vi "ExperimentLoop.vi"(8 "Error In":errorcluster, 9 "ABLE Configuration":T1, 10 "ABLE Data Structures":T7, 11 "Action Queues":T8) -> (0 "Error Out":errorcluster)   [LabVIEW 2012]
uses:
  ActionQueues.ctl
  UIActionQueueElement.ctl
  UIAction.ctl
  HardwareActionQueueElement.ctl
  HardwareAction.ctl
  ExperimentActionQueueElement.ctl
  ExperimentAction.ctl
  AlarmQueueElement.ctl
  AlarmAction.ctl
  ABLEDataStructures.ctl
  HardwareDisplayData.ctl
  BPM.ctl
  ExperimentHardwareData.ctl
  ExperimentData.ctl
  AlarmData.ctl
  AlarmDatum.ctl
  ABLEConfiguration.ctl
  DisplayConfiguration.ctl
  FolderConfiguration.ctl
  AlarmsConfiguration.ctl
  Keithley6485Configuration.ctl
  Keithley6482Configuration.ctl
  Experiment.ctl
  Sample.ctl
  BeamLine.ctl
  BeamLineType.ctl
  BeamLineIon.ctl
  ExperimentRun.ctl
  ExperimentRunTiming.ctl
  ExperimentRunDose.ctl
  ExperimentRunFluence.ctl
  ExperimentRunTotalCharge.ctl
  ExperimentLogActionQueueElement.ctl
  ExperimentLogAction.ctl
  ExperimentLogData.ctl
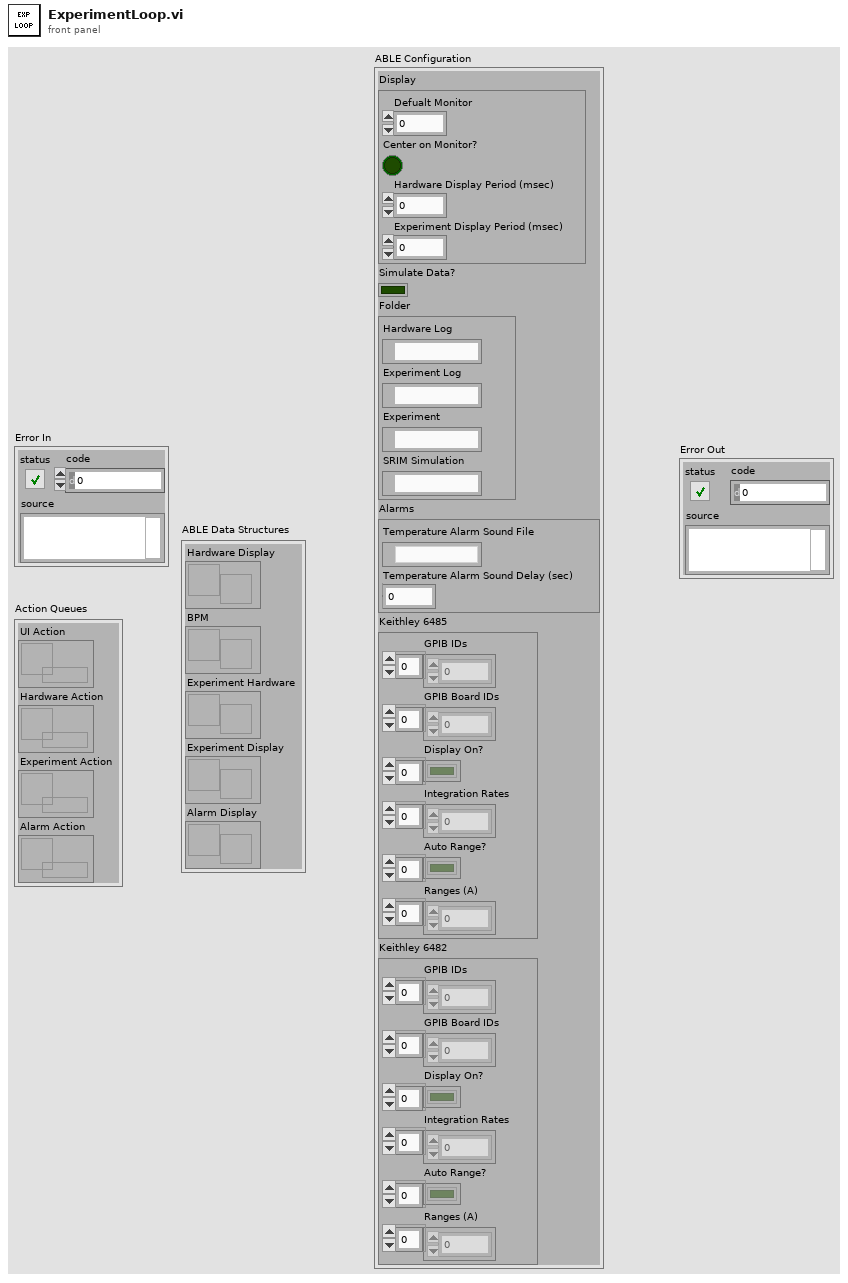
[diagram p1: front panel]
types:
  T1 = typedef "ABLEConfiguration.ctl" = cluster{"Display":T2, "Simulate Data?":bool, "Folder":T3, "Alarms":T4, "Keithley 6485":T5, "Keithley 6482":T6}
  T2 = typedef "DisplayConfiguration.ctl" = cluster{"Defualt Monitor":u16, "Center on Monitor?":bool, "Hardware Display Period (msec)":u32, "Experiment Display Period (msec)":u32}
  T3 = typedef "FolderConfiguration.ctl" = cluster{"Hardware Log":path, "Experiment Log":path, "Experiment":path, "SRIM Simulation":path}
  T4 = typedef "AlarmsConfiguration.ctl" = cluster{"Temperature Alarm Sound File":path, "Temperature Alarm Sound Delay (sec)":dbl}
  T5 = typedef "Keithley6485Configuration.ctl" = cluster{"GPIB IDs":u8[], "GPIB Board IDs":u8[], "Display On?":bool[], "Integration Rates":dbl[], "Auto Range?":bool[], "Ranges (A)":dbl[]}
  T6 = typedef "Keithley6482Configuration.ctl" = cluster{"GPIB IDs":u8[], "GPIB Board IDs":u8[], "Display On?":bool[], "Integration Rates":dbl[], "Auto Range?":bool[], "Ranges (A)":dbl[]}
  T7 = typedef "ABLEDataStructures.ctl" = cluster{"Hardware Display":refnum<notifier>, "BPM":refnum<notifier>, "Experiment Hardware":refnum<notifier>, "Experiment Display":refnum<notifier>, "Alarm Display":refnum<notifier>}
  T8 = typedef "ActionQueues.ctl" = cluster{"UI Action":refnum<queue>, "Hardware Action":refnum<queue>, "Experiment Action":refnum<queue>, "Alarm Action":refnum<queue>}
  T9 = typedef "Experiment.ctl" = cluster{"File Path":path, "Operator":string, "Project":string, "Target Dose (dpa)":dbl, "Sample":T10, "Beam Line":T11, "Runs":T14[]}
  T10 = typedef "Sample.ctl" = cluster{"Name":string, "Description":string, "Molar Mass (g/mol)":dbl, "Density (g/cm^3)":dbl, "Irradiation Area (cm^2)":dbl, "SRIM Damage Peak (disp * ions/cm)":dbl}
  T11 = typedef "BeamLine.ctl" = cluster{"Type":T12, "Ion":T13, "Charge State":u8, "Total Source Ion Energy (kV)":dbl}
  T12 = typedef "BeamLineType.ctl" = enum16{"Ion Beam Analysis", "Auxiliary", "Radiation Damage"}
  T13 = typedef "BeamLineIon.ctl" = enum16{"H", "He", "C", "Fe", "Ni", "Pt", "Si", "Ag", "Au"}
  T14 = typedef "ExperimentRun.ctl" = cluster{"Timing":T15, "Dose (dpa)":T16, "Fluence (ions/cm^2)":T17, "Total Charge (C)":T18}
  T15 = typedef "ExperimentRunTiming.ctl" = cluster{"Start":timestamp, "Stop":timestamp}
  T16 = typedef "ExperimentRunDose.ctl" = cluster{"Start":dbl, "Stop":dbl}
  T17 = typedef "ExperimentRunFluence.ctl" = cluster{"Start":dbl, "Stop":dbl}
  T18 = typedef "ExperimentRunTotalCharge.ctl" = cluster{"Start":dbl, "Stop":dbl}
  T19 = typedef "ExperimentLogData.ctl" = cluster{"Time Stamp":timestamp, "Experiment Data":T20}
  T20 = typedef "ExperimentData.ctl" = cluster{"Flux (ions/s * cm^2)":dbl, "Average Flux (ions/s * cm^2)":dbl, "DPA Rate":dbl, "Average DPA Rate":dbl, "Total Ion Energy (MeV)":dbl, "Total Charge (C)":dbl, "Dose (DPA)":dbl, "Fluence (ions/cm^2)":dbl, "Percent Complete (%)":dbl, "Duration (sec)":dbl}
  T21 = typedef "ExperimentLogActionQueueElement.ctl" = cluster{"Action":T22, "Data":variant}
  T22 = typedef "ExperimentLogAction.ctl" = enum16{"Initialize", "Clear", "Create", "Log", "Stop", "Shutdown"}
  T23 = typedef "UIActionQueueElement.ctl" = cluster{"Action":T24, "Data":variant}
  T24 = typedef "UIAction.ctl" = enum16{"Initalize", "Create Experiment", "Created", "Read Experiment Controls", "Read Alarm Controls", "Loaded", "Save Experiment", "Saved", "Write Experiment Controls", "Read Experiment", "Read", "Start Experiment", "Started", "Stop Experiment", "Stopped", "Close Experiment", "Closed", "SRIM", "Error", "Shutdown"}
  T25 = typedef "ExperimentActionQueueElement.ctl" = cluster{"Action":T26, "Data":variant}
  T26 = typedef "ExperimentAction.ctl" = enum16{"Initialize", "Create", "Read", "Load", "Start", "Run", "Stop", "Save", "Shutdown"}
  T27 = typedef "ExperimentHardwareData.ctl" = cluster{"Beam Current (A)":dbl, "Terminal Voltage (MeV)":dbl}
  T28 = cluster{"seconds since 1Jan1904":timestamp, "Total Charge Out (C)":dbl, "Total Charge Out (C)":dbl, "Total Charge Out (C)":dbl}
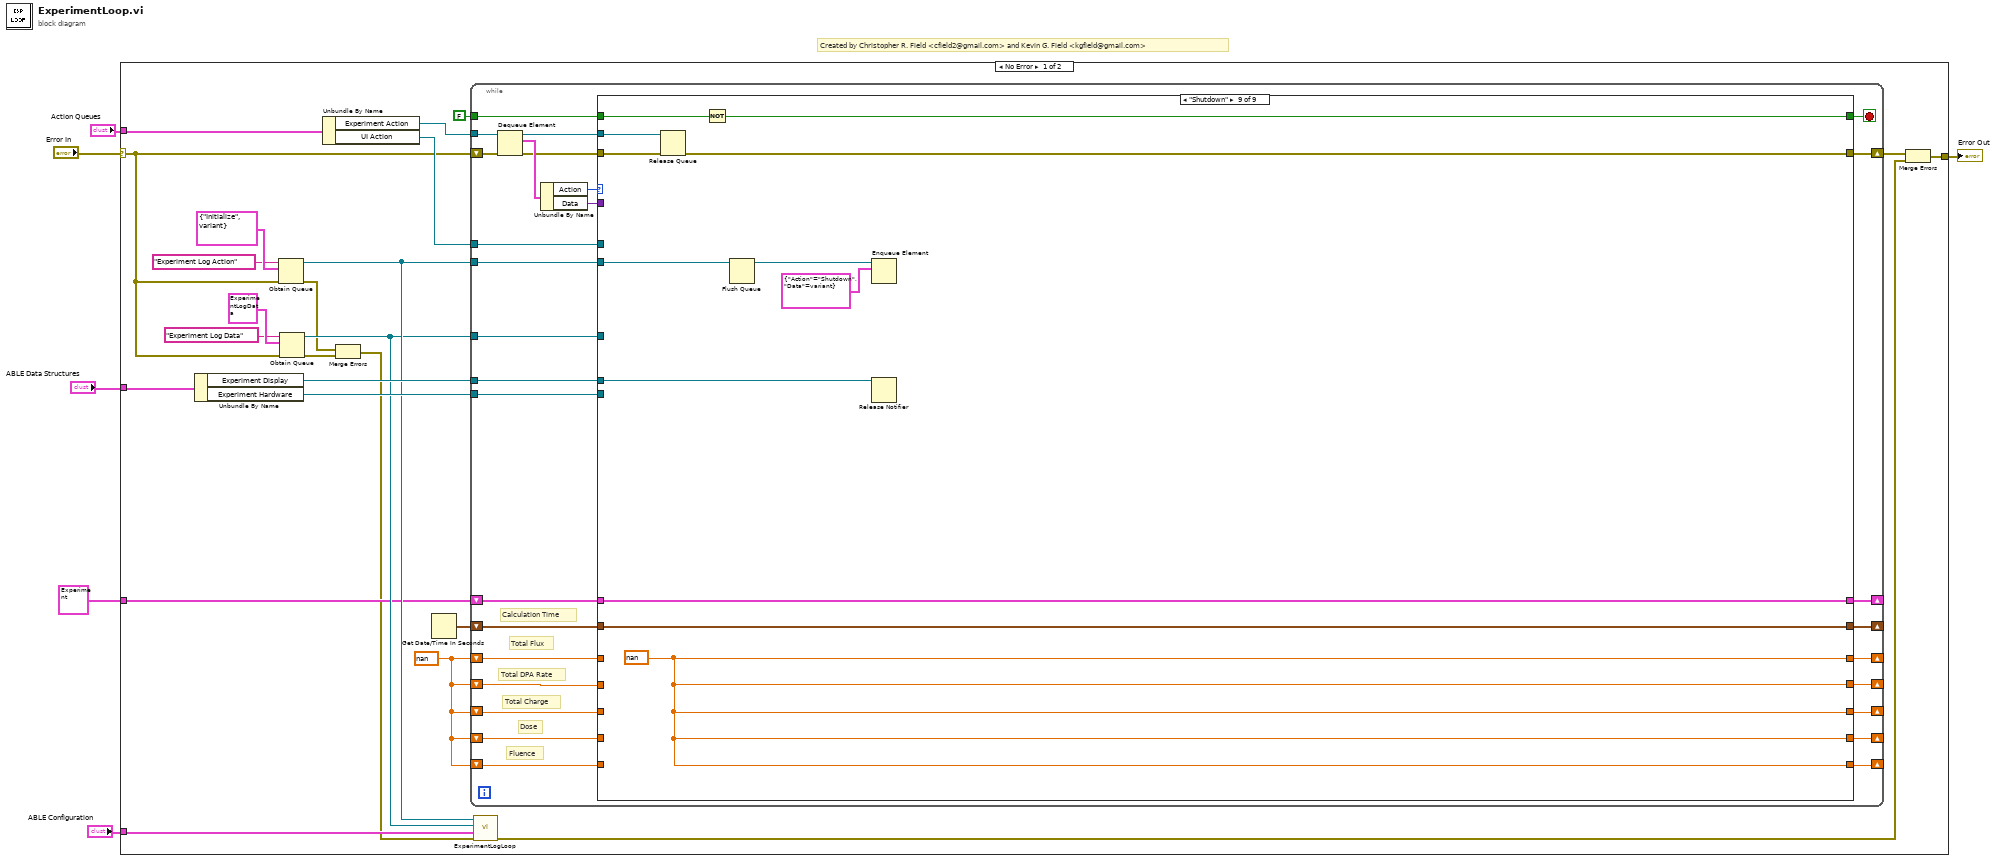
[diagram p0: block diagram]
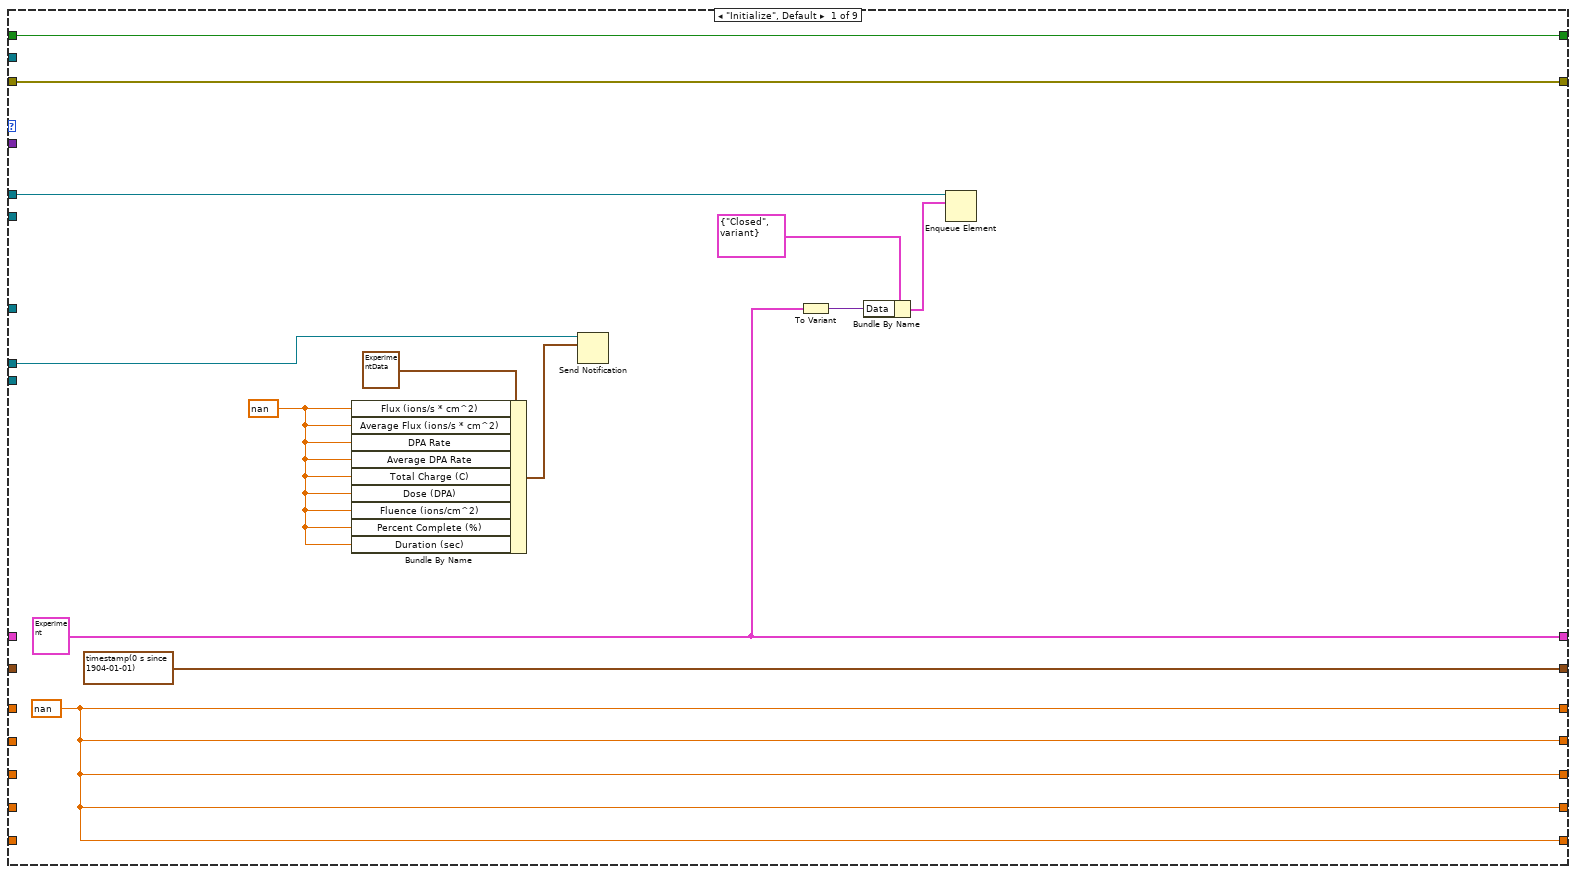
[diagram p2: hidden frame]
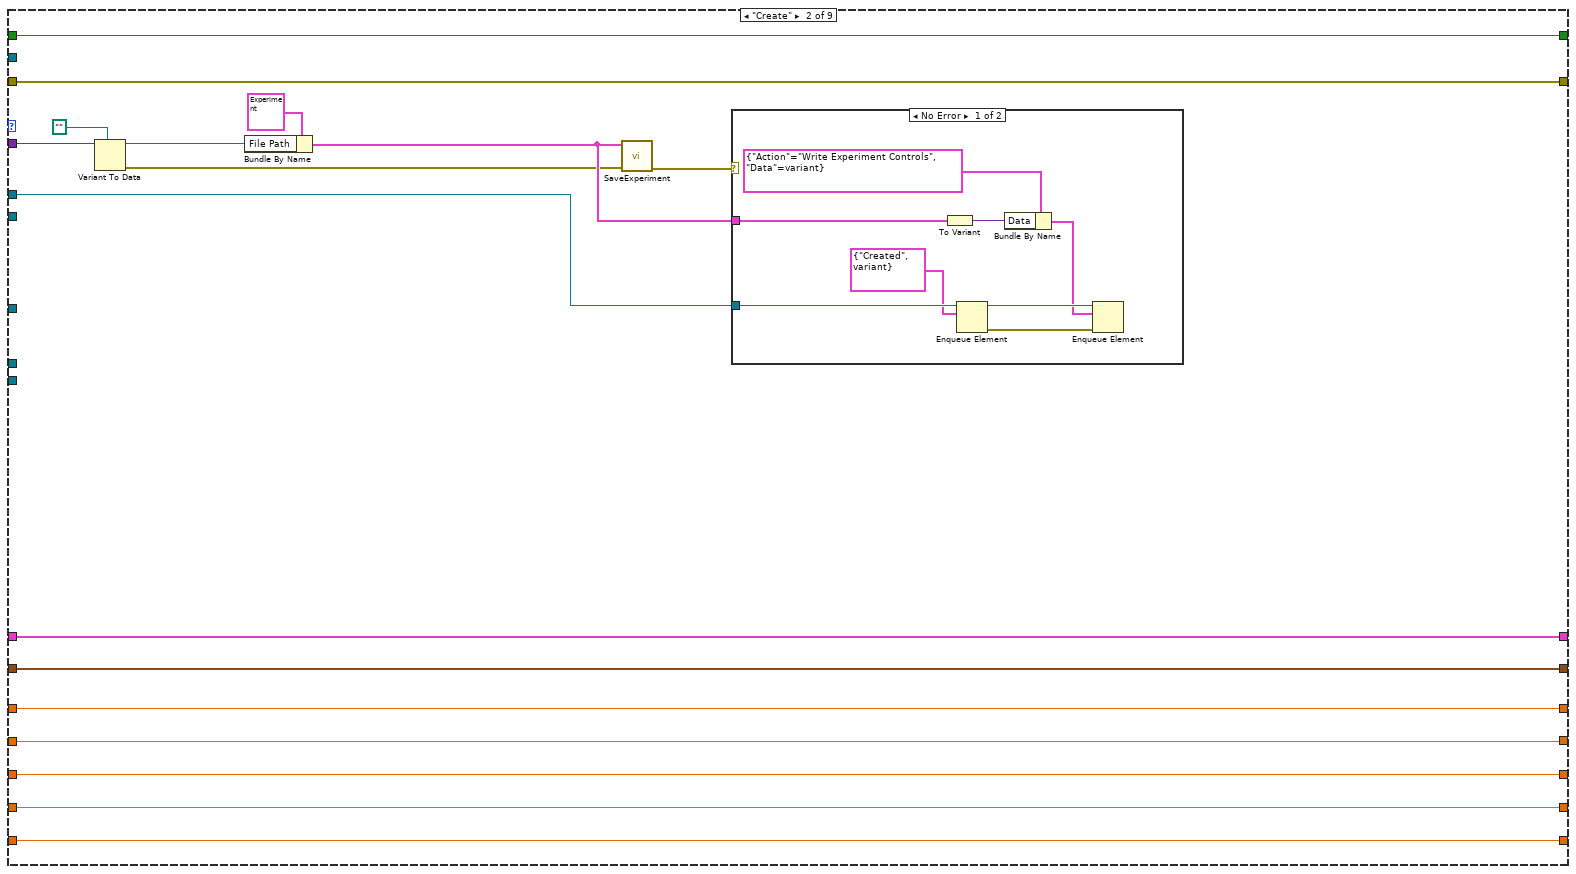
[diagram p3: hidden frame]
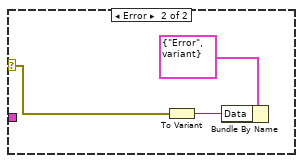
[diagram p4: hidden frame]
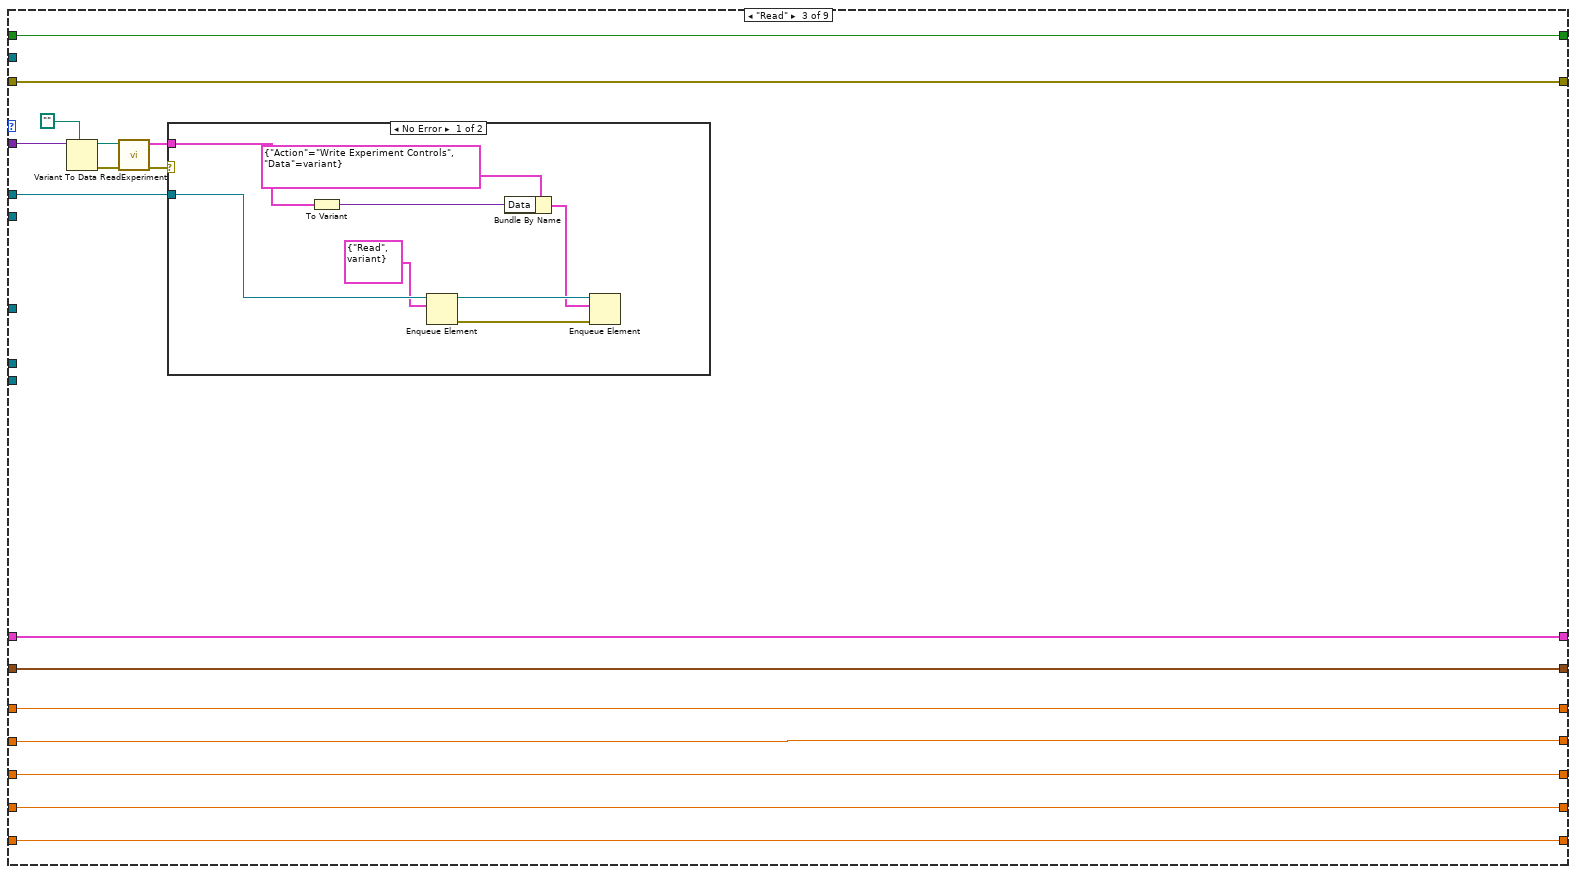
[diagram p5: hidden frame]
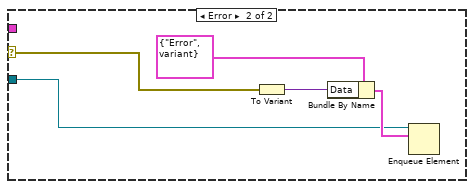
[diagram p6: hidden frame]
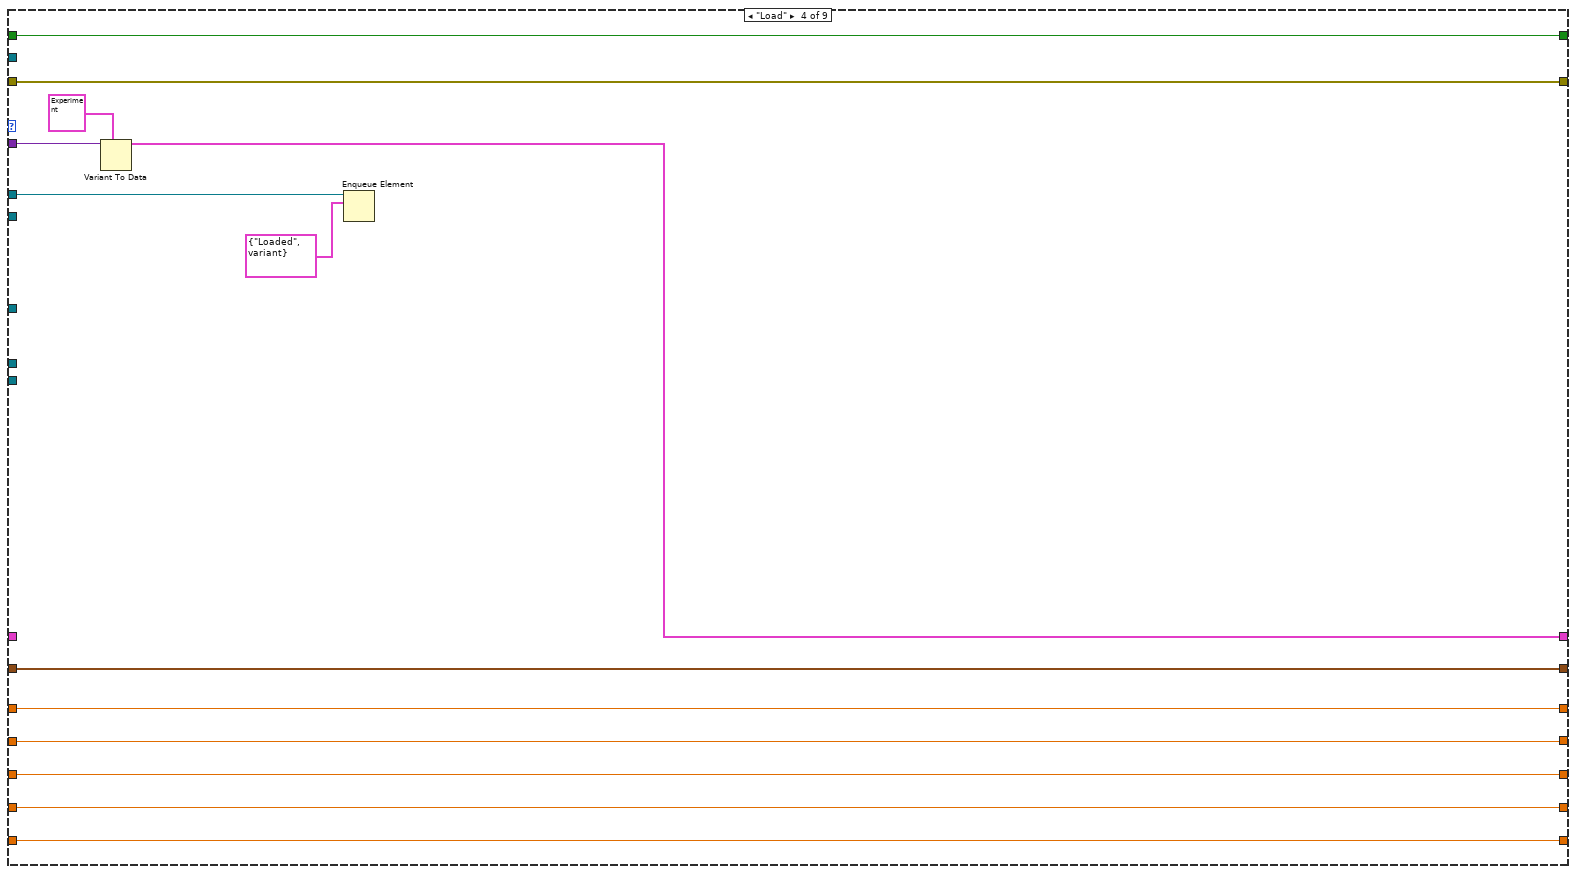
[diagram p7: hidden frame]
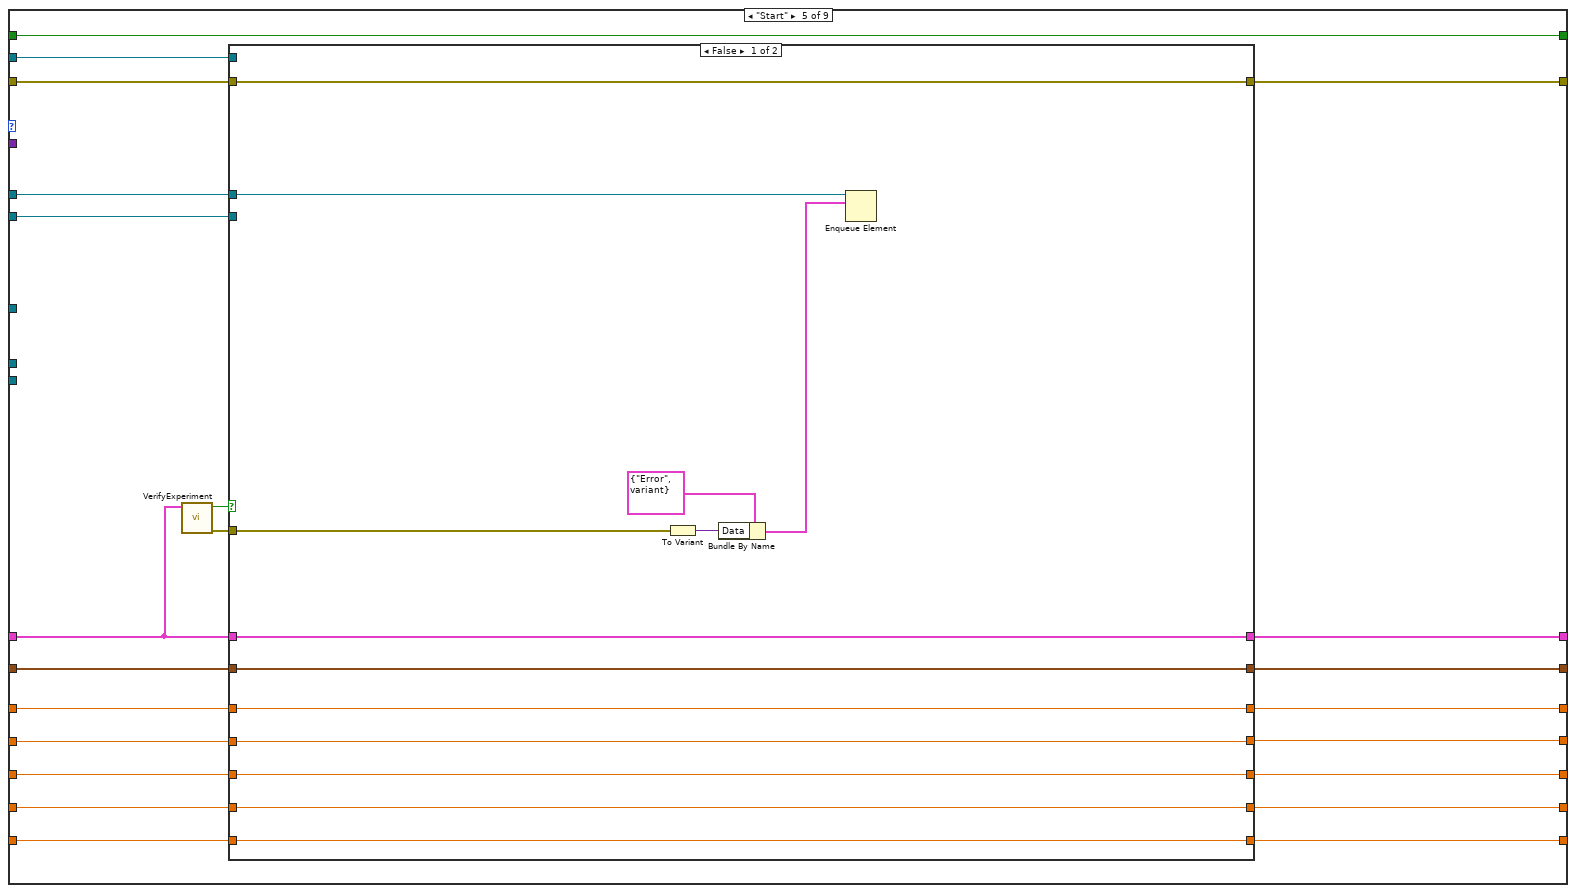
[diagram p8: hidden frame]
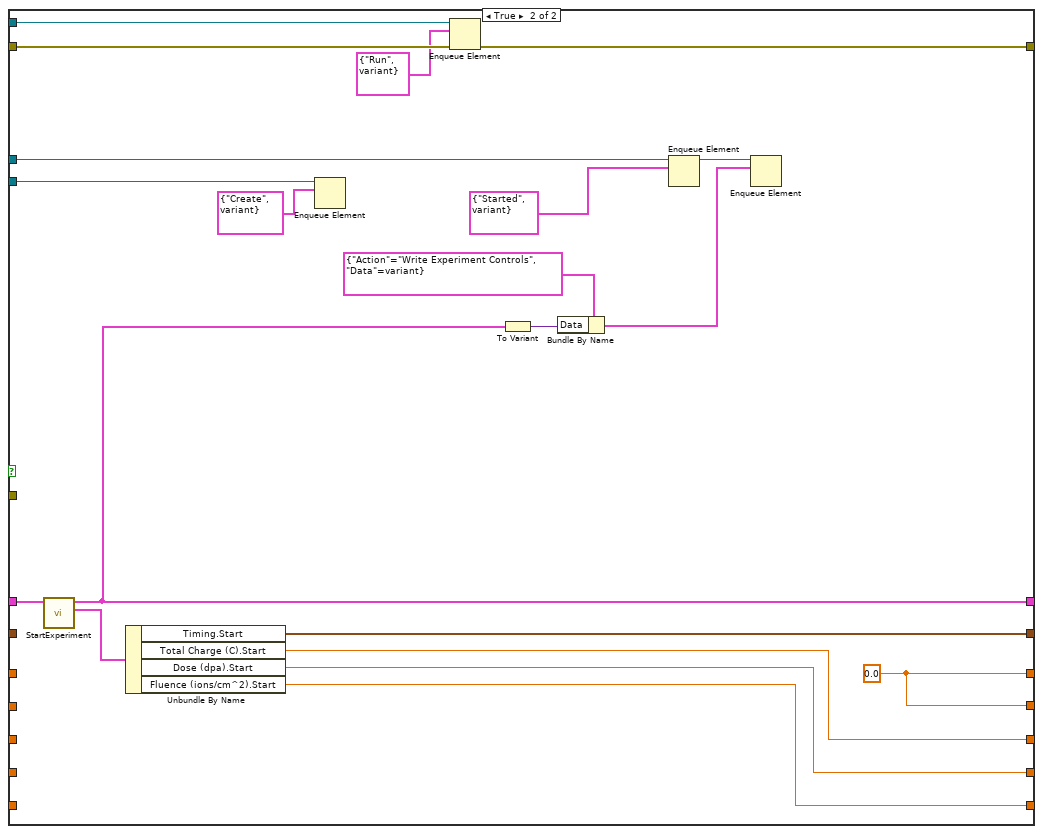
[diagram p9: hidden frame]
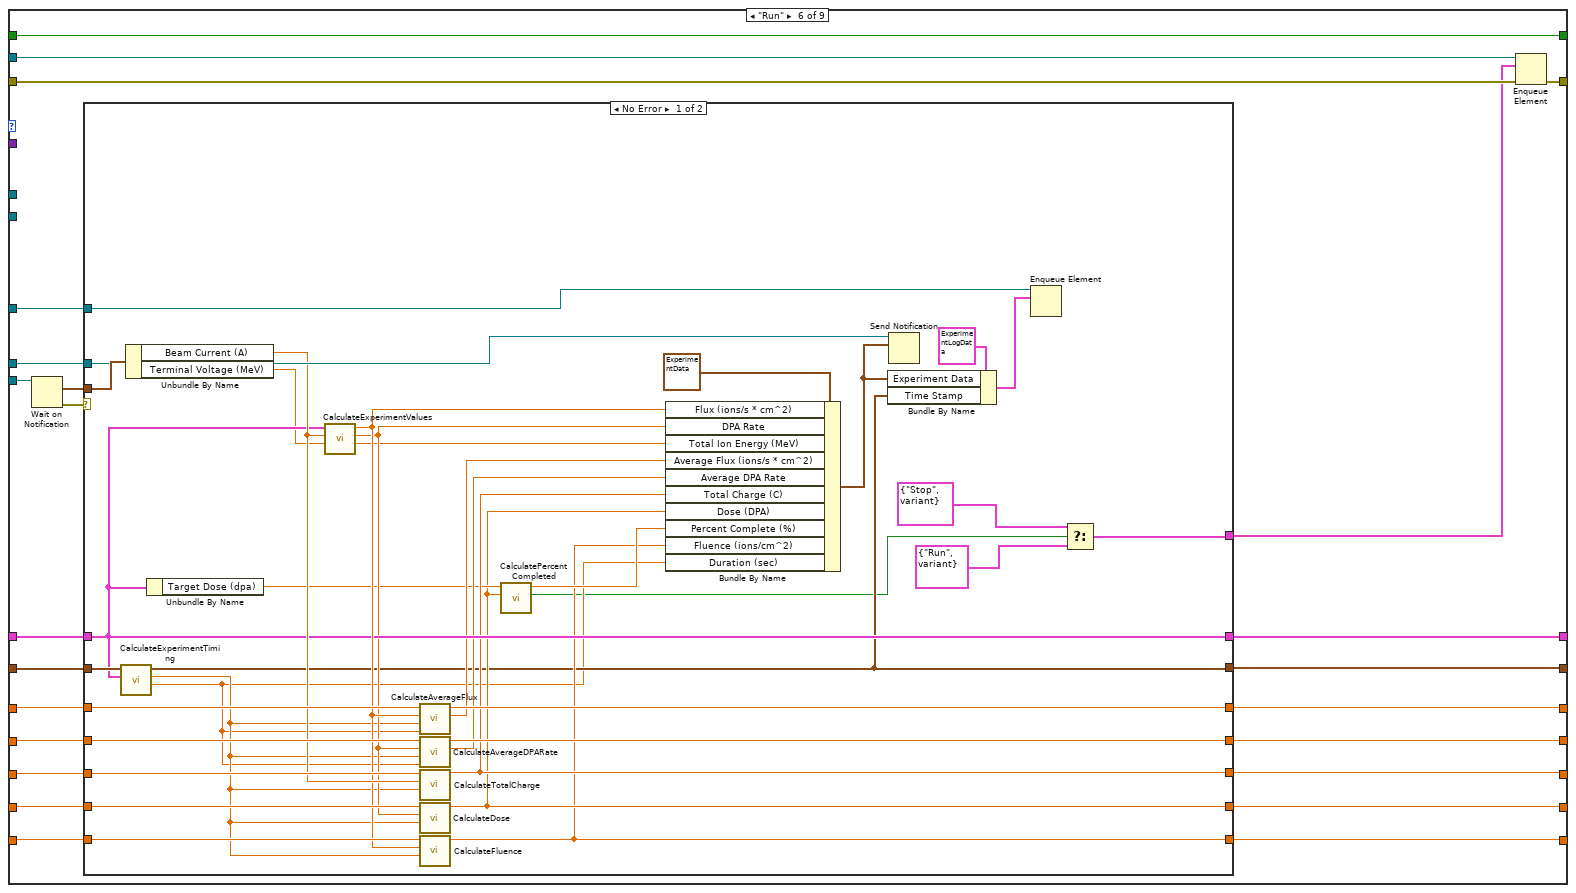
[diagram p10: hidden frame]
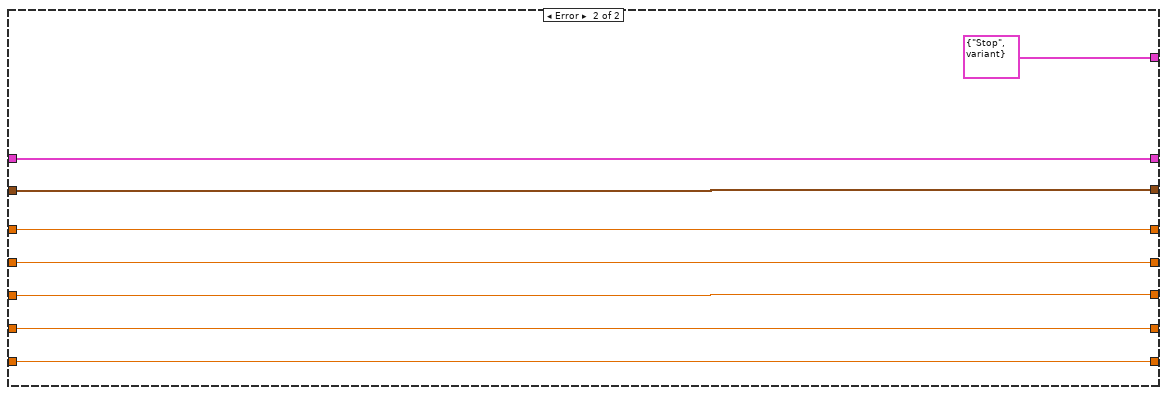
[diagram p11: hidden frame]
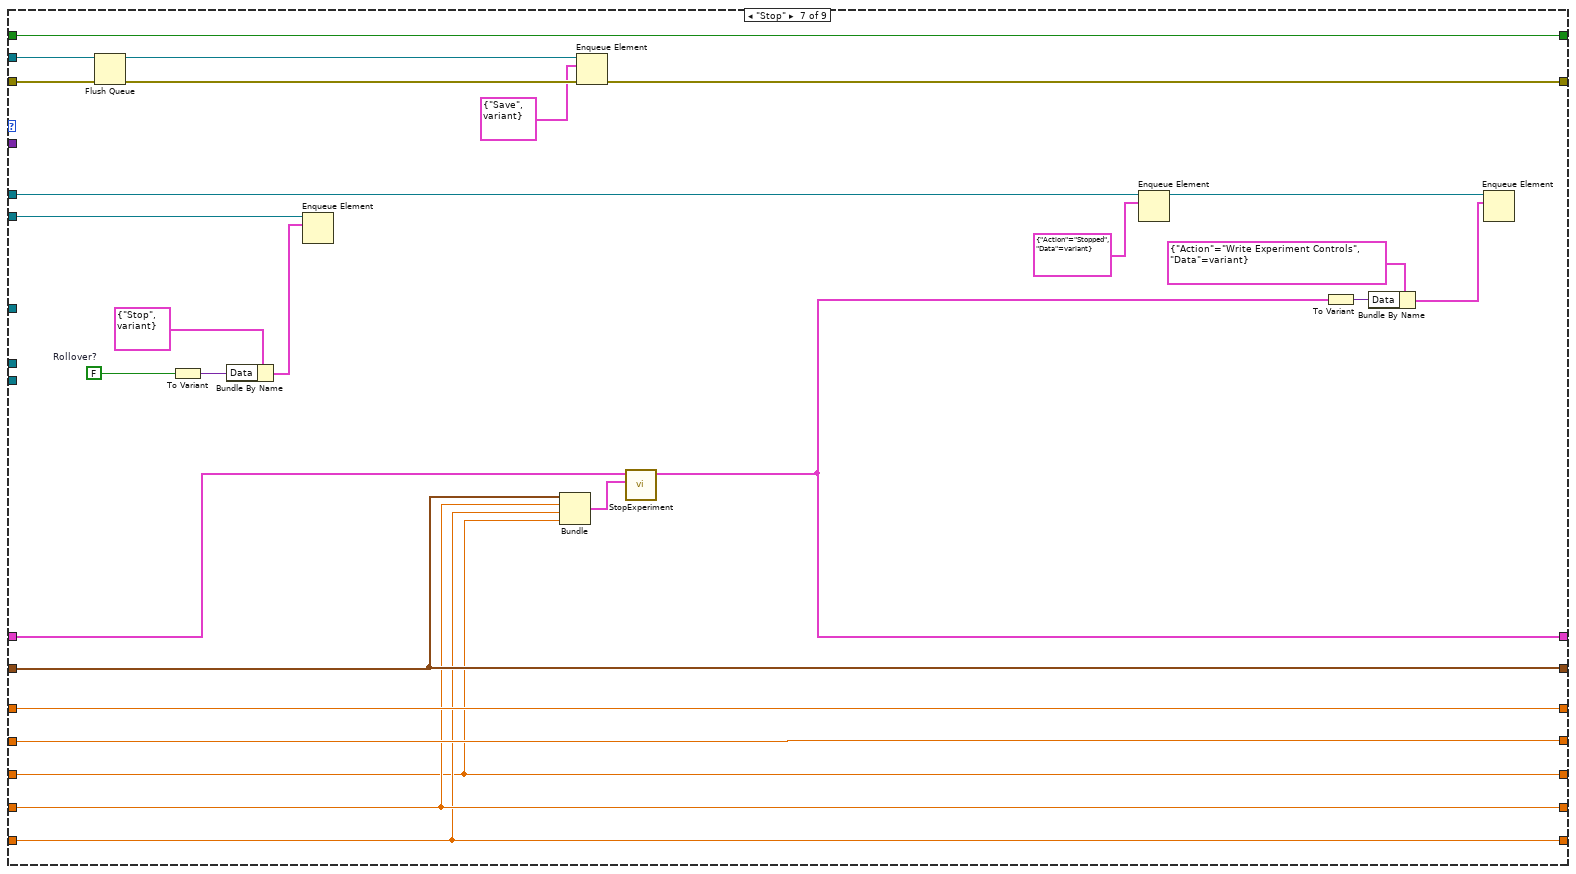
[diagram p12: hidden frame]
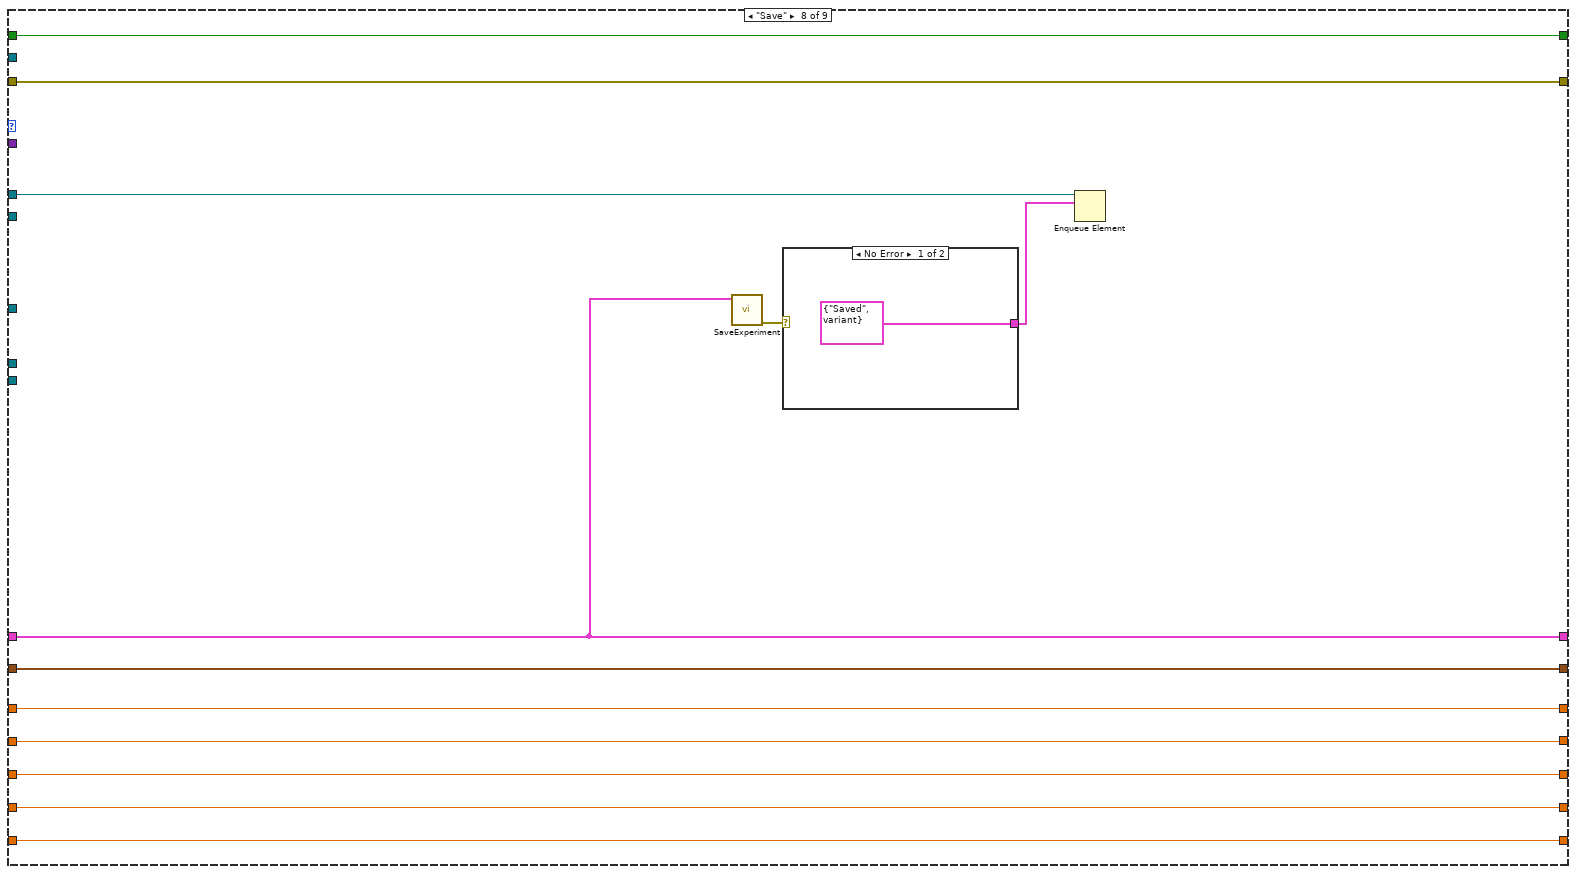
[diagram p13: hidden frame]
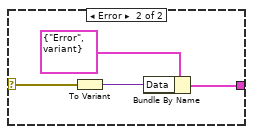
[diagram p14: hidden frame]
diagram:
  # "Created by Christopher R. Field <cfield2@gmail.com> and Kevin G. Field <kgfield@gmail.com>"
  n1 = case shown="No Error" "Error In" {
    selector: "Error In" -> [w10 w321]
    tunnel: "Action Queues" -> [w29 _]
    tunnel: [w13 w321] -> w5
    tunnel: "ABLE Data Structures" -> [w27 _]
    tunnel: T9 {"File Path"=path "", "Operator"="Operator", "Project"="Project Description", "Target Dose (dpa)"=nan, "Sample"={"Name"="Sample Name", "Description"="Sample Description", "Molar Mass (g/mol)"=nan, "Density (g/cm^3)"=nan, "Irradiation Area (cm^2)"=nan, "SRIM Damage Peak (disp * ions/cm)"=nan}, "Beam Line"={"Type"=enum."Ion Beam Analysis", "Ion"=enum."H", "Charge State"=0, "Total Source Ion Energy (kV)"=nan}, "Runs"=[]} ("Experiment Configuration") -> [w11 _]
    tunnel: "ABLE Configuration" -> [w15 _]
    frame No Error {
      w23 = nan ("Total Charge Out (C)")
      n2 = Unbundle By Name(w27) -> ("Experiment Display"=w24:refnum<notifier>, "Experiment Hardware"=w26:refnum<notifier>)
      n3 = Obtain Queue(name (unnamed)="Experiment Log Action", element data type=T21 {"Action"=enum."Initialize", "Data"=variant} ("Experiment Log Action Queue Element"), error in (no error)=w10) -> (queue out=w17:refnum<queue>, error out=w8:errorcluster)  [unwired: 2 in, 1 out]
      n4 = Obtain Queue(name (unnamed)="Experiment Log Data", element data type=T19 {"Time Stamp"=timestamp(0 s since 1904-01-01), "Experiment Data"={"Flux (ions/s * cm^2)"=0.0, "Average Flux (ions/s * cm^2)"=0.0, "DPA Rate"=0.0, "Average DPA Rate"=0.0, "Total Ion Energy (MeV)"=0.0, "Total Charge (C)"=0.0, "Dose (DPA)"=0.0, "Fluence (ions/cm^2)"=0.0, "Percent Complete (%)"=0.0, "Duration (sec)"=0.0}} ("Experiment Log Data"), error in (no error)=w10) -> (queue out=w16:refnum<queue>, error out=w9:errorcluster)  [unwired: 2 in, 1 out]
      n5 = Unbundle By Name(w29) -> ("Experiment Action"=w28:refnum<queue>, "UI Action"=w22:refnum<queue>)
      n6 = Merge Errors(w8, w9) -> (w7:errorcluster)
      n7 = Get Date/Time In Seconds() -> (seconds since 1Jan1904=w25:timestamp)
      n8 = while {
        tunnel: FALSE -> [w51]
        tunnel: w28 -> [w58]
        shift-right: [w52] -> w14
        shift-left: w10 -> [w59]
        shift-right: [w48] -> _
        shift-left: w25 -> [w49]
        shift-right: [w47] -> _
        shift-left: w23 -> [w46]
        shift-right: [w45] -> _
        shift-left: w23 -> [w44]
        shift-right: [w43] -> _
        shift-left: w23 -> [w42]
        shift-right: [w40] -> _
        shift-left: w23 -> [w41]
        shift-right: [w38] -> _
        shift-left: w23 -> [w39]
        tunnel: w26 -> [w37]
        tunnel: w24 -> [w36]
        shift-right: [w34] -> _
        shift-left: w11 -> [w35]
        tunnel: w22 -> [w33]
        tunnel: w17 -> [w31]
        tunnel: w16 -> [w32]
        stop <- w50 stop-if-true
        # "Calculation Time"
        # "Total DPA Rate"
        # "Total Flux"
        # "Dose"
        # "Fluence"
        # "Total Charge"
        n9 = Dequeue Element(queue=w58, error in (no error)=w59) -> (queue out=w53:refnum<queue>, element=w57:T25, error out=w54:errorcluster)  [unwired: 1 in, 1 out]
        n10 = Unbundle By Name(w57) -> ("Action"=w56:T26, "Data"=w55:variant)
        n11 = case shown="\"Shutdown\"" w56 {
          tunnel: w55 -> [_ w86 w116 w140 _ _ _ _ _]
          tunnel: w54 -> [w71 w88 w113 w141 w162 w208 w287 w302 w315]
          tunnel: w53 -> [_ _ _ _ w163 w209 w288 _ w316]
          tunnel: [w71 w88 w113 w141 w161 w207 w283 w302 w314] -> w52
          tunnel: w51 -> [w72 w89 w114 w142 w164 w221 w291 w303 w320]
          tunnel: [w72 w89 w114 w142 w164 w221 w291 w303 w319] -> w50
          tunnel: w49 -> [_ w82 w107 w137 w150 w220 w269 w301 w318]
          tunnel: [timestamp(0 s since 1904-01-01) ("seconds since 1Jan1904") w82 w107 w137 w153 w218 w269 w301 w318] -> w48
          tunnel: [w65 w79 w110 w134 w156 w204 w266 w298 w312] -> w47
          tunnel: w46 -> [_ w79 w110 w134 w147 w219 w266 w298 _]
          tunnel: [w65 w78 w109 w133 w155 w203 w268 w297 w312] -> w45
          tunnel: w44 -> [_ w78 w109 w133 w146 w211 w268 w297 _]
          tunnel: [w65 w77 w108 w132 w154 w202 w267 w296 w312] -> w43
          tunnel: w42 -> [_ w77 w108 w132 w145 w210 w267 w296 _]
          tunnel: w41 -> [_ w80 w111 w135 w148 w214 w290 w299 _]
          tunnel: [w65 w80 w111 w135 w144 w212 w290 w299 w312] -> w40
          tunnel: w39 -> [_ w81 w112 w136 w149 w215 w277 w300 _]
          tunnel: [w65 w81 w112 w136 w158 w213 w277 w300 w312] -> w38
          tunnel: w37 -> [_ _ _ _ _ w217 _ _ _]
          tunnel: w36 -> [w69 _ _ _ _ w206 _ _ w311]
          tunnel: w35 -> [_ w83 w102 _ w151 w205 w271 w295 w317]
          tunnel: [w60 w83 w102 w138 w157 w198 w270 w295 w317] -> w34
          tunnel: w33 -> [w64 w73 w101 w131 w160 _ w289 w294 _]
          tunnel: w32 -> [_ _ _ _ _ w199 _ _ _]
          tunnel: w31 -> [_ _ _ _ w159 _ w286 _ w310]
          frame "Initialize", Default {
            w65 = nan ("Total Charge Out (C)")
            w60 = T9 {"File Path"=path "", "Operator"="Operator", "Project"="Project Description", "Target Dose (dpa)"=nan, "Sample"={"Name"="Sample Name", "Description"="Sample Description", "Molar Mass (g/mol)"=nan, "Density (g/cm^3)"=nan, "Irradiation Area (cm^2)"=nan, "SRIM Damage Peak (disp * ions/cm)"=nan}, "Beam Line"={"Type"=enum."Ion Beam Analysis", "Ion"=enum."H", "Charge State"=1, "Total Source Ion Energy (kV)"=nan}, "Runs"=[]} ("Experiment Configuration")
            w67 = nan ("Flux (ions/s * cm^2)")
            n12 = Bundle By Name(cluster=T20 {"Flux (ions/s * cm^2)"=0.0, "Average Flux (ions/s * cm^2)"=0.0, "DPA Rate"=0.0, "Average DPA Rate"=0.0, "Total Ion Energy (MeV)"=0.0, "Total Charge (C)"=0.0, "Dose (DPA)"=0.0, "Fluence (ions/cm^2)"=0.0, "Percent Complete (%)"=0.0, "Duration (sec)"=0.0} ("Experiment Data"), "Flux (ions/s * cm^2)"=w67, "Average Flux (ions/s * cm^2)"=w67, "DPA Rate"=w67, "Average DPA Rate"=w67, "Total Charge (C)"=w67, "Dose (DPA)"=w67, "Fluence (ions/cm^2)"=w67, "Percent Complete (%)"=w67, "Duration (sec)"=w67) -> (w68:T20)
            n13 = Send Notification(notification=w68, notifier=w69) -> ()  [unwired: 1 in, 2 out]
            n14 = To Variant(anything=w60) -> (Variant=w61:variant)
            n15 = Bundle By Name(cluster=T23 {"Action"=enum."Closed", "Data"=variant} ("element"), "Data"=w61) -> (w62:T23)
            n16 = Enqueue Element(queue=w64, element=w62) -> ()  [unwired: 2 in, 3 out]
          }
          frame "Create" {
            n17 = Variant To Data(type=path "", Variant=w86) -> (data=w84:path, error out=w74:errorcluster)  [unwired: 1 in]
            n18 = Bundle By Name(cluster=T9 {"File Path"=path "", "Operator"="Operator", "Project"="Project Description", "Target Dose (dpa)"=0.0, "Sample"={"Name"="Sample Name", "Description"="Sample Description", "Molar Mass (g/mol)"=0.0, "Density (g/cm^3)"=0.0, "Irradiation Area (cm^2)"=0.0, "SRIM Damage Peak (disp * ions/cm)"=0.0}, "Beam Line"={"Type"=enum."Ion Beam Analysis", "Ion"=enum."H", "Charge State"=1, "Total Source Ion Energy (kV)"=0.0}, "Runs"=[]} ("Experiment Configuration"), "File Path"=w84) -> (w75:T9)
            n19 = call "SaveExperiment.vi"("Error In"=w74, "Experiment"=w75) -> ("Error Out"=w76:errorcluster)  [unwired: 9 in]
            n20 = case shown="No Error" w76 {
              selector: w76 -> [_ w98]
              tunnel: w75 -> [w96 _]
              tunnel: w73 -> [w95 _]
              frame No Error {
                n21 = To Variant(anything=w96) -> (Variant=w97:variant)
                n22 = Enqueue Element(queue=w95, element=T23 {"Action"=enum."Created", "Data"=variant}) -> (queue out=w93:refnum<queue>, error out=w90:errorcluster)  [unwired: 2 in, 1 out]
                n23 = Bundle By Name(cluster=T23 {"Action"=enum."Write Experiment Controls", "Data"=variant} ("element"), "Data"=w97) -> (w91:T23)
                n24 = Enqueue Element(queue=w93, element=w91, error in (no error)=w90) -> ()  [unwired: 1 in, 3 out]
              }
              frame Error {
                n25 = To Variant(anything=w98) -> (Variant=w99:variant)
                n26 = Bundle By Name(cluster=T23 {"Action"=enum."Error", "Data"=variant} ("element"), "Data"=w99) -> ()  [unwired: 1 out]
              }
            }
          }
          frame "Read" {
            n27 = Variant To Data(type=path "", Variant=w116) -> (data=w106:path, error out=w105:errorcluster)  [unwired: 1 in]
            n28 = call "ReadExperiment.vi"("Error In"=w105, "Experiment File Path"=w106) -> ("Error Out"=w104:errorcluster, "Experiment"=w103:T9)  [unwired: 8 in]
            n29 = case shown="No Error" w104 {
              selector: w104 -> [_ w125]
              tunnel: w103 -> [w122 _]
              tunnel: w101 -> [w121 w126]
              frame No Error {
                n30 = To Variant(anything=w122) -> (Variant=w123:variant)
                n31 = Enqueue Element(queue=w121, element=T23 {"Action"=enum."Read", "Data"=variant}) -> (queue out=w119:refnum<queue>, error out=w117:errorcluster)  [unwired: 2 in, 1 out]
                n32 = Bundle By Name(cluster=T23 {"Action"=enum."Write Experiment Controls", "Data"=variant} ("element"), "Data"=w123) -> (w118:T23)
                n33 = Enqueue Element(queue=w119, element=w118, error in (no error)=w117) -> ()  [unwired: 1 in, 3 out]
              }
              frame Error {
                n34 = To Variant(anything=w125) -> (Variant=w128:variant)
                n35 = Bundle By Name(cluster=T23 {"Action"=enum."Error", "Data"=variant} ("element"), "Data"=w128) -> (w127:T23)
                n36 = Enqueue Element(queue=w126, element=w127) -> ()  [unwired: 2 in, 3 out]
              }
            }
          }
          frame "Load" {
            n37 = Variant To Data(type=T9 {"File Path"=path "", "Operator"="Operator", "Project"="Project Description", "Target Dose (dpa)"=0.0, "Sample"={"Name"="", "Description"="", "Molar Mass (g/mol)"=0.0, "Density (g/cm^3)"=0.0, "Irradiation Area (cm^2)"=0.0, "SRIM Damage Peak (disp * ions/cm)"=0.0}, "Beam Line"={"Type"=enum."Ion Beam Analysis", "Ion"=enum."H", "Charge State"=0, "Total Source Ion Energy (kV)"=nan}, "Runs"=[]} ("Experiment"), Variant=w140) -> (data=w138:T9)  [unwired: 1 in, 1 out]
            n38 = Enqueue Element(queue=w131, element=T23 {"Action"=enum."Loaded", "Data"=variant}) -> ()  [unwired: 2 in, 3 out]
          }
          frame "Start" {
            n39 = call "VerifyExperiment.vi"("Experiment"=w151) -> ("Error Out"=w143:errorcluster, "Experiment Valid?"=w152:bool)  [unwired: 9 in]
            n40 = case shown="False" w152 {
              tunnel: w163 -> [_ w197]
              tunnel: w162 -> [w177 w196]
              tunnel: [w177 w195] -> w161
              tunnel: w160 -> [w169 w193]
              tunnel: w159 -> [_ w192]
              tunnel: [w174 w184] -> w158
              tunnel: [w176 w182] -> w157
              tunnel: [w172 w189] -> w156
              tunnel: [w171 w188] -> w155
              tunnel: [w170 w187] -> w154
              tunnel: [w175 w186] -> w153
              tunnel: w151 -> [w176 w185]
              tunnel: w150 -> [w175 _]
              tunnel: w149 -> [w174 _]
              tunnel: w148 -> [w173 _]
              tunnel: w147 -> [w172 _]
              tunnel: w146 -> [w171 _]
              tunnel: w145 -> [w170 _]
              tunnel: [w173 w184] -> w144
              tunnel: w143 -> [w165 _]
              frame False {
                n41 = To Variant(anything=w165) -> (Variant=w167:variant)
                n42 = Bundle By Name(cluster=T23 {"Action"=enum."Error", "Data"=variant} ("element"), "Data"=w167) -> (w166:T23)
                n43 = Enqueue Element(queue=w169, element=w166) -> ()  [unwired: 2 in, 3 out]
              }
              frame True {
                w184 = 0.0 ("Total Charge Out (C)")
                n44 = call "StartExperiment.vi"("Experiment In"=w185) -> ("Experiment Run"=w190:T14, "Experiment Out"=w182:T9)  [unwired: 9 in]
                n45 = Unbundle By Name(w190) -> ("Timing.Start"=w186:timestamp, "Total Charge (C).Start"=w189:dbl, "Dose (dpa).Start"=w188:dbl, "Fluence (ions/cm^2).Start"=w187:dbl)
                n46 = Enqueue Element(queue=w192, element=T21 {"Action"=enum."Create", "Data"=variant}) -> ()  [unwired: 2 in, 3 out]
                n47 = Enqueue Element(queue=w197, element=T25 {"Action"=enum."Run", "Data"=variant}, error in (no error)=w196) -> (error out=w195:errorcluster)  [unwired: 1 in, 2 out]
                n48 = To Variant(anything=w182) -> (Variant=w183:variant)
                n49 = Bundle By Name(cluster=T23 {"Action"=enum."Write Experiment Controls", "Data"=variant} ("element"), "Data"=w183) -> (w178:T23)
                n50 = Enqueue Element(queue=w193, element=T23 {"Action"=enum."Started", "Data"=variant}) -> (queue out=w179:refnum<queue>)  [unwired: 2 in, 2 out]
                n51 = Enqueue Element(queue=w179, element=w178) -> ()  [unwired: 2 in, 3 out]
              }
            }
          }
          frame "Run" {
            n52 = Wait on Notification(notifier=w217) -> (notification=w216:T27, error out=w201:errorcluster)  [unwired: 3 in, 2 out]
            n53 = case shown="No Error" w201 {
              tunnel: w220 -> [w237 w259]
              tunnel: w219 -> [w256 w262]
              tunnel: [w224 w259] -> w218
              tunnel: w216 -> [w255 _]
              tunnel: w215 -> [w253 w264]
              tunnel: w214 -> [w252 w263]
              tunnel: [w251 w264] -> w213
              tunnel: [w250 w263] -> w212
              tunnel: w211 -> [w249 w261]
              tunnel: w210 -> [w248 w260]
              tunnel: w206 -> [w247 _]
              tunnel: w205 -> [w236 w257]
              tunnel: [w230 w262] -> w204
              tunnel: [w228 w261] -> w203
              tunnel: [w226 w260] -> w202
              tunnel: [w242 T25 {"Action"=enum."Stop", "Data"=variant} ("element")] -> w200
              tunnel: w199 -> [w239 _]
              tunnel: [w236 w257] -> w198
              frame No Error {
                n54 = call "CalculateExperimentTiming.vi"("Experiment"=w236, "Calculation Start Time In"=w237) -> ("Duration (sec)"=w223:dbl, "Period (sec)"=w225:dbl, "Calculation Start Time Out"=w224:timestamp)  [unwired: 7 in]
                n55 = Unbundle By Name(w255) -> ("Beam Current (A)"=w246:dbl, "Terminal Voltage (MeV)"=w235:dbl)
                n56 = Unbundle By Name(w236) -> ("Target Dose (dpa)"=w229:dbl)
                n57 = call "CalculateExperimentValues.vi"("Terminal Voltage (V)"=w235, "Beam Current (A)"=w246, "Experiment"=w236) -> ("Total Ion Energy (MeV)"=w233:dbl, "DPA Rate"=w234:dbl, "Flux (ions/s * cm^2)"=w245:dbl)  [unwired: 5 in, 1 out]
                n58 = call "CalculateAverageFlux.vi"("Duration"=w223, "Period"=w225, "Flux"=w245, "Total Flux In"=w253) -> ("Average Flux"=w232:dbl, "Total Flux Out"=w251:dbl)  [unwired: 6 in]
                n59 = call "CalculateAverageDPARate.vi"("Duration (sec)"=w223, "Period (sec)"=w225, "DPA Rate"=w234, "Total DPA Rate In"=w252) -> ("Average DPA Rate"=w231:dbl, "Total DPA Rate Out"=w250:dbl)  [unwired: 6 in]
                n60 = call "CalculateTotalCharge.vi"("Period (sec)"=w225, "Beam Current (A)"=w246, "Total Charge In (C)"=w256) -> ("Total Charge Out (C)"=w230:dbl)  [unwired: 8 in]
                n61 = call "CalculateDose.vi"("Period (sec)"=w225, "DPA Rate"=w234, "Dose In (DPA)"=w249) -> ("Dose Out (DPA)"=w228:dbl)  [unwired: 8 in]
                n62 = call "CalculateFluence.vi"("Period (s)"=w225, "Flux (ions/s * cm^2)"=w245, "Fluence In (ions/cm^2)"=w248) -> ("Fluence Out (ions/cm^2)"=w226:dbl)  [unwired: 8 in]
                n63 = call "CalculatePercentCompleted.vi"("Dose (dpa)"=w228, "Target Dose (dpa)"=w229) -> ("Complete?"=w222:bool, "Percent Complete (%)"=w227:dbl)  [unwired: 8 in]
                n64 = Bundle By Name(cluster=T20 {"Flux (ions/s * cm^2)"=0.0, "Average Flux (ions/s * cm^2)"=0.0, "DPA Rate"=0.0, "Average DPA Rate"=0.0, "Total Ion Energy (MeV)"=0.0, "Total Charge (C)"=0.0, "Dose (DPA)"=0.0, "Fluence (ions/cm^2)"=0.0, "Percent Complete (%)"=0.0, "Duration (sec)"=0.0} ("Experiment Data"), "Flux (ions/s * cm^2)"=w245, "DPA Rate"=w234, "Total Ion Energy (MeV)"=w233, "Average Flux (ions/s * cm^2)"=w232, "Average DPA Rate"=w231, "Total Charge (C)"=w230, "Dose (DPA)"=w228, "Percent Complete (%)"=w227, "Fluence (ions/cm^2)"=w226, "Duration (sec)"=w223) -> (w240:T20)
                n65 = Bundle By Name(cluster=T19 {"Time Stamp"=timestamp(0 s since 1904-01-01), "Experiment Data"={"Flux (ions/s * cm^2)"=0.0, "Average Flux (ions/s * cm^2)"=0.0, "DPA Rate"=0.0, "Average DPA Rate"=0.0, "Total Ion Energy (MeV)"=0.0, "Total Charge (C)"=0.0, "Dose (DPA)"=0.0, "Fluence (ions/cm^2)"=0.0, "Percent Complete (%)"=0.0, "Duration (sec)"=0.0}} ("Experiment Log Data"), "Experiment Data"=w240, "Time Stamp"=w224) -> (w238:T19)
                n66 = Send Notification(notification=w240, notifier=w247) -> ()  [unwired: 1 in, 2 out]
                n67 = Enqueue Element(queue=w239, element=w238) -> ()  [unwired: 2 in, 3 out]
                n68 = Select(t=T25 {"Action"=enum."Stop", "Data"=variant} ("element"), s=w222, f=T25 {"Action"=enum."Run", "Data"=variant} ("element")) -> (s? t:f=w242:T25)
              }
              frame Error {
              }
            }
            n69 = Enqueue Element(queue=w209, element=w200, error in (no error)=w208) -> (error out=w207:errorcluster)  [unwired: 1 in, 2 out]
          }
          frame "Stop" {
            w279 = FALSE  # Rollover?
            n70 = Flush Queue(queue=w288, error in (no error)=w287) -> (queue out=w285:refnum<queue>, error out=w284:errorcluster)  [unwired: 1 out]
            n71 = To Variant(anything=w279) -> (Variant=w278:variant)
            n72 = Bundle By Name(cluster=T21 {"Action"=enum."Stop", "Data"=variant} ("element"), "Data"=w278) -> (w280:T21)
            n73 = Enqueue Element(queue=w286, element=w280) -> ()  [unwired: 2 in, 3 out]
            n74 = Bundle("seconds since 1Jan1904"=w269, "Total Charge Out (C)"=w268, "Total Charge Out (C)"=w267, "Total Charge Out (C)"=w266) -> (w265:T28)  [unwired: 1 in]
            n75 = Enqueue Element(queue=w285, element=T25 {"Action"=enum."Save", "Data"=variant}, error in (no error)=w284) -> (error out=w283:errorcluster)  [unwired: 1 in, 2 out]
            n76 = call "StopExperiment.vi"("Stop Values"=w265, "Experiment In"=w271) -> ("Experiment Out"=w270:T9)  [unwired: 9 in]
            n77 = Enqueue Element(queue=w289, element=T23 {"Action"=enum."Stopped", "Data"=variant}) -> (queue out=w273:refnum<queue>)  [unwired: 2 in, 2 out]
            n78 = To Variant(anything=w270) -> (Variant=w275:variant)
            n79 = Bundle By Name(cluster=T23 {"Action"=enum."Write Experiment Controls", "Data"=variant} ("element"), "Data"=w275) -> (w274:T23)
            n80 = Enqueue Element(queue=w273, element=w274) -> ()  [unwired: 2 in, 3 out]
          }
          frame "Save" {
            n81 = call "SaveExperiment.vi"("Experiment"=w295) -> ("Error Out"=w293:errorcluster)  [unwired: 10 in]
            n82 = case shown="No Error" w293 {
              selector: w293 -> [_ w305]
              tunnel: [T23 {"Action"=enum."Saved", "Data"=variant} ("element") w307] -> w292
              frame No Error {
              }
              frame Error {
                n83 = To Variant(anything=w305) -> (Variant=w306:variant)
                n84 = Bundle By Name(cluster=T23 {"Action"=enum."Error", "Data"=variant} ("element"), "Data"=w306) -> (w307:T23)
              }
            }
            n85 = Enqueue Element(queue=w294, element=w292) -> ()  [unwired: 2 in, 3 out]
          }
          frame "Shutdown" {
            w312 = nan ("Total Charge Out (C)")
            n86 = Release Queue(queue=w316, error in (no error)=w315) -> (error out=w314:errorcluster)  [unwired: 1 in, 2 out]
            n87 = Not(x=w320) -> (.not. x?=w319:bool)
            n88 = Flush Queue(queue=w310) -> (queue out=w309:refnum<queue>)  [unwired: 1 in, 2 out]
            n89 = Release Notifier(notifier=w311) -> ()  [unwired: 2 in, 3 out]
            n90 = Enqueue Element(queue=w309, element=T21 {"Action"=enum."Shutdown", "Data"=variant}) -> ()  [unwired: 2 in, 3 out]
          }
        }
      }
      n91 = call "ExperimentLogLoop.vi"("Error In"=w7, "ABLE Configuration"=w15, "Experiment Log Data"=w16, "Experiment Log Action Queue"=w17) -> ("Error Out"=w12:errorcluster)  [unwired: 7 in]
      n92 = Merge Errors(w14, w12) -> (w13:errorcluster)
    }
    frame Error {
    }
  }
  "Error Out" <- w5
